vi "testCameraNetworkController.vi"() -> ()   [LabVIEW 2009, in "run.lvlib"]
uses:
  testing/run.lvlib
  Tools/Filing/FileSystem/FileSystem.lvclass
  CameraNetworkController.lvclass
  Tools/Filing/FileNeologist/FileNeologist.lvclass
panel:
  in  "number of Images":i32=-1
  in  "remote port":u16=6340
  in  "remote address":string="192.168.104.187"
  out "stopped?":bool
  in  "stop":bool
  in  "saveImages?":bool
  in  "camera":string
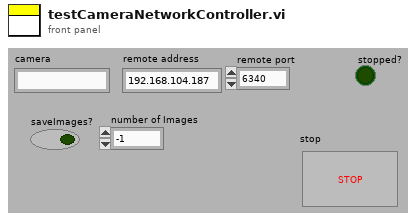
[diagram p1: front panel]
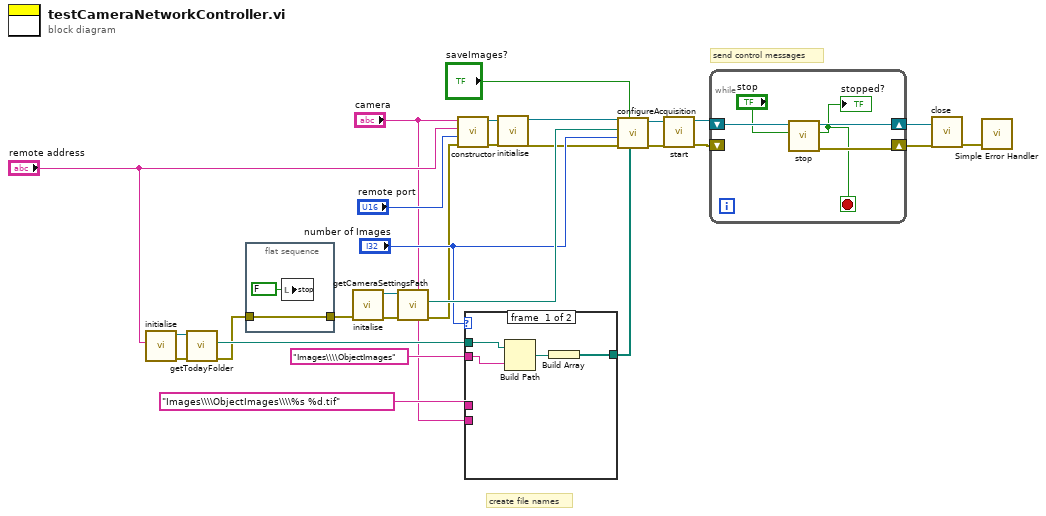
[diagram p0: block diagram]
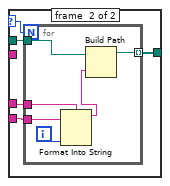
[diagram p2: hidden frame]
diagram:
  # "send control messages"
  # "create file names"
  n1 = call "initialise.vi"("computer name"="remote address") -> ("error out"=w15:errorcluster, "FileNeologist out"=w16:refnum<class "FileNeologist.lvclass">)  [unwired: 9 in]
  n2 = call "getTodayFolder.vi"("error in (no error)"=w15, "FileNeologist in"=w16) -> ("error out"=w20:errorcluster, "todayFolder"=w28:path)  [unwired: 7 in, 1 out]
  n3 = flat-sequence {
    tunnel: w20 -> [w30]
    tunnel: [w30] -> w19
    frame #0 {
      n4 = local write "stop"(FALSE) -> ()
    }
  }
  n5 = call "initalise.vi"("error in (no error)"=w19) -> ("error out"=w25:errorcluster, "FileSystem out"=w26:refnum<class "FileSystem.lvclass">)  [unwired: 9 in]
  n6 = call-dynamic "getCameraSettingsPath.vi"("error in (no error)"=w25, "FileSystem.lvclass in"=w26) -> ("error out"=w17:errorcluster, "CameraSettingsPath"=w24:path)  [unwired: 7 in, 1 out]
  n7 = call "constructor.vi"("error in (no error)"=w17, "remote port"="remote port", "remote address"="remote address", "camera"="camera") -> ("error out"=w12:errorcluster, "CameraNetworkController out"=w5:refnum<class "CameraNetworkController.lvclass">)  [unwired: 6 in]
  n8 = case shown="1, Default" "number of Images" {
    selector: "number of Images" -> [_ w36]
    tunnel: w28 -> [w33 w39]
    tunnel: [w34 w38] -> w23
    tunnel: "Images\\\\ObjectImages\\\\%s %d.tif" -> [_ w37]
    tunnel: "camera" -> [_ w35]
    tunnel: "Images\\\\ObjectImages" -> [w32 _]
    frame #0 {
      n9 = Build Path(base path=w33, name or relative path=w32) -> (appended path=w31:path)
      n10 = Build Array(w31) -> (w34:path[])
    }
    frame #1 {
      n11 = for {
        N: w36 -> [_]
        tunnel: w39 -> [w45]
        tunnel: [w44] -> w38 mode=indexing
        tunnel: w37 -> [w43]
        tunnel: w35 -> [w41]
        i -> [w42]
        n12 = Format Into String(format string=w43, w41, w42) -> (resulting string=w40:string)  [unwired: 2 in, 1 out]
        n13 = Build Path(base path=w45, name or relative path=w40) -> (appended path=w44:path)
      }
    }
  }
  n14 = call "initialise.vi"("error in (no error)"=w12, "CameraNetworkController in"=w5) -> ("error out"=w10:errorcluster, "CameraNetworkController out"=w11:refnum<class "CameraNetworkController.lvclass">)  [unwired: 8 in]
  n15 = call "configureAcquisition.vi"("imagePaths"=w23, "save?"="saveImages?", "error in (no error)"=w10, "numberImages"="number of Images", "settingsPath"=w24, "CameraNetworkController in"=w11) -> ("error out"=w7:errorcluster, "CameraNetworkController out"=w8:refnum<class "CameraNetworkController.lvclass">)  [unwired: 4 in]
  n16 = call "start.vi"("error in (no error)"=w7, "CameraNetworkController in"=w8) -> ("error out"=w3:errorcluster, "CameraNetworkController out"=w4:refnum<class "CameraNetworkController.lvclass">)  [unwired: 8 in]
  n17 = while {
    shift-right: [w49] -> w6
    shift-left: w4 -> [w50]
    shift-right: [w48] -> w2
    shift-left: w3 -> [_]
    stop <- w46 stop-if-true
    n18 = call "stop.vi"("stop"="stop", "CameraNetworkController in"=w50) -> ("error out"=w48:errorcluster, "stopped?"=w46:bool, "CameraNetworkController out"=w49:refnum<class "CameraNetworkController.lvclass">)  [unwired: 7 in]
    "stopped?" <- w46
  }
  n19 = call "close.vi"("error in (no error)"=w2, "CameraNetworkController in"=w6) -> ("error out"=w1:errorcluster)  [unwired: 8 in, 1 out]
  n20 = call <vilib>:"Simple Error Handler.vi"("error in (no error)"=w1) -> ()  [unwired: 4 in, 5 out]
